vi "TSCAN DBCAnalysisTransmit.vi"(0 "路径输入":path, 1 "Message":string, 2 "Signal":string, 3 "SigValue":dbl, 11 "错误输入（无错误）":errorcluster) -> (4 "路径输出":path, 6 "FData":T1, 15 "错误输出":errorcluster)   [LabVIEW 2013]
panel:
  in  "簇":T2
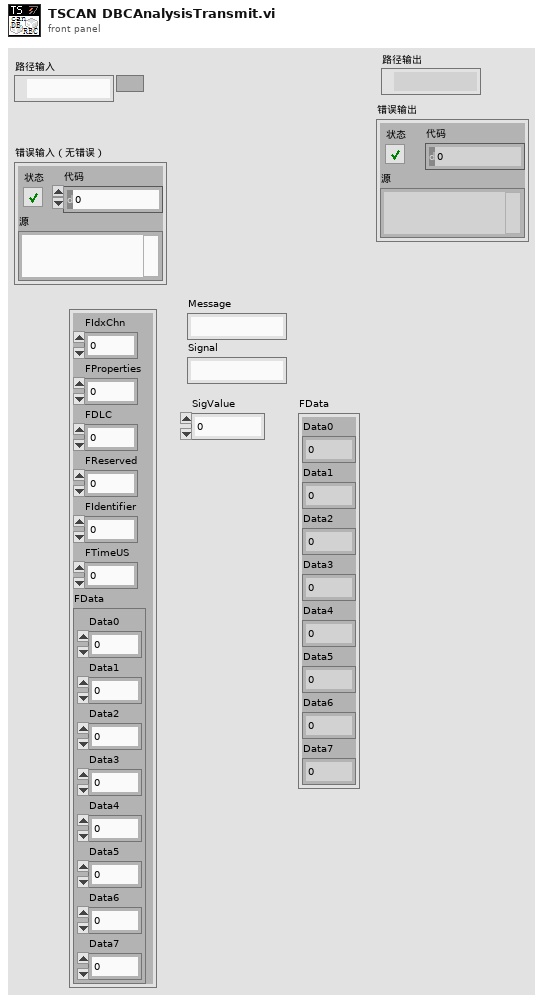
[diagram p1: front panel]
types:
  T1 = cluster{"Data0":u8, "Data1":u8, "Data2":u8, "Data3":u8, "Data4":u8, "Data5":u8, "Data6":u8, "Data7":u8}
  T2 = cluster{"FIdxChn":u8, "FProperties":u8, "FDLC":u8, "FReserved":u8, "FIdentifier":i32, "FTimeUS":u64, "FData":cluster{"Data0":u8, "Data1":u8, "Data2":u8, "Data3":u8, "Data4":u8, "Data5":u8, "Data6":u8, "Data7":u8}}
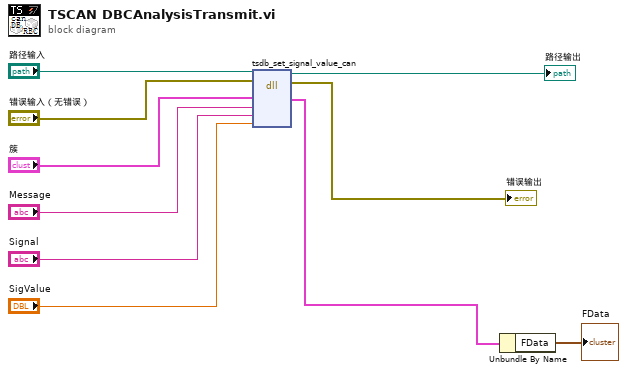
[diagram p0: block diagram]
diagram:
  n1 = dll-call lib="PTH17abs EDemo同星\nTSCAN_V1.0ConfigTSMaster.dll" fn="tsdb_set_signal_value_can"(path in="路径输入", error in="错误输入（无错误）", "CANObJ"="簇", "Message"="Message", "Signal"="Signal", "SigValue"="SigValue") -> (path out=→"路径输出":path, error out=→"错误输出":errorcluster, "CANObJ"=w2:T2)  [unwired: 5 in]
  n2 = Unbundle By Name(w2) -> ("FData"=→"FData":T1)
